vi "Algae Command_wrapper.vi"() -> ()   [LabVIEW 2023]
uses:
  Implementation/Algae Operations.ctl
  Support Code/Teleop Util/Algae States.ctl
  <vilib>/Rock Robotics/WPI/Framework/Completion Status.ctl
  <vilib>/Rock Robotics/WPI/Framework/Completion Notifier.ctl
  <vilib>/Rock Robotics/WPI/Framework/Command Status Info.ctl
panel:
  out "Command Info Out":T1
  in  "Command Info In":T1
  in  "Negate or Confirm?":bool
  in  "Description":string
  in  "Setpoint":dbl
  in  "Algae State":T4=enum."Intake Algae"
  in  "Operation":T5
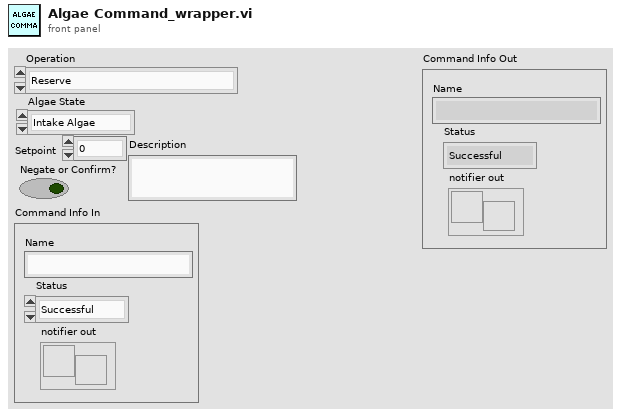
[diagram p1: front panel]
types:
  T1 = typedef "Command Status Info.ctl" = cluster{"Name":string, "Status":T2, "notifier out":T3}
  T2 = typedef "Completion Status.ctl" = enum16{"Successful", "Aborted", "Incomplete"}
  T3 = typedef "Completion Notifier.ctl" = refnum<notifier>
  T4 = typedef "Algae States.ctl" = enum16{"Idle", "Intake Algae", "Outtake Algae", "Stow", "Manual Overrides"}
  T5 = typedef "Algae Operations.ctl" = enum16{"Reserve", "Read Current", "Immediate", "Calibrate"}
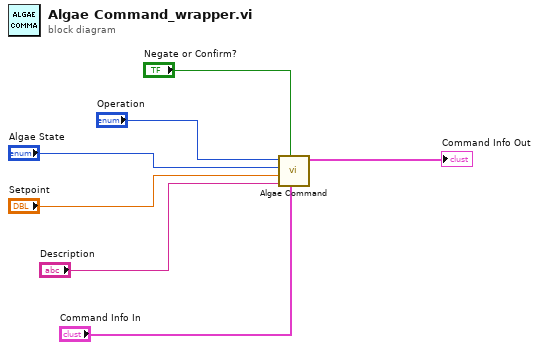
[diagram p0: block diagram]
diagram:
  n1 = call "Algae Command.vi"("Command Info In"="Command Info In", "Negate or Confirm?"="Negate or Confirm?", "Description"="Description", "Setpoint"="Setpoint", "Algae State"="Algae State", "Operation"="Operation") -> ("Command Info Out"=→"Command Info Out":T1)  [unwired: 5 in]
